vi "Check if Attribute is a Pointer.vi"(7 "Test ID":string, 8 "error in (no error)":errorcluster, 9 "Type":variant, 10 "Attribute Name":string, 11 "Test Executive in":refnum<class "Test Executive.lvclass">) -> (0 "error out":errorcluster, 1 "Pointer ID":string, 2 "Pointer?":bool, 3 "Test Executive out":refnum<class "Test Executive.lvclass">, 4 "Pointer Attribute Name":string)   [LabVIEW 2019, in "Test Executive.lvlib" / "Test Executive.lvclass"]
uses:
  <vilib>/gpm_packages/@cs/test-executive/Source/Test Executive/TestExecutive/Test Executive.lvclass
  <vilib>/gpm_packages/@cs/test-executive/Source/Test Executive/TestExecutive/Test Executive.lvclass/Test Executive.ctl
  67b02e64-984f-4c06-84dc-e4ea2e0dd7a9.vi
  <vilib>/gpm_packages/@cs/linked-list/Source/Linked List/ILinkedList/ILinked List.lvclass
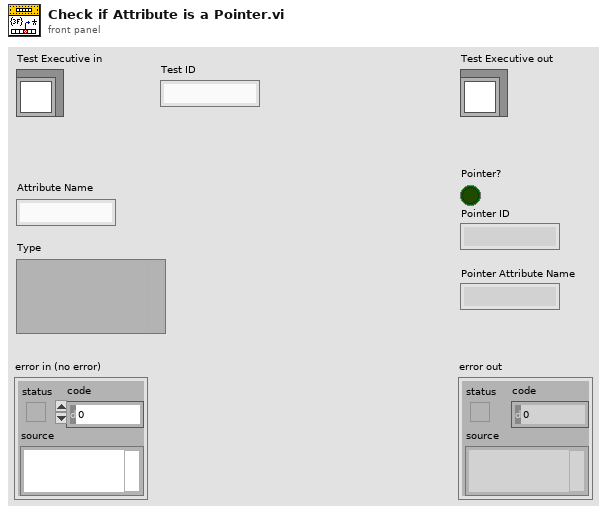
[diagram p1: front panel]
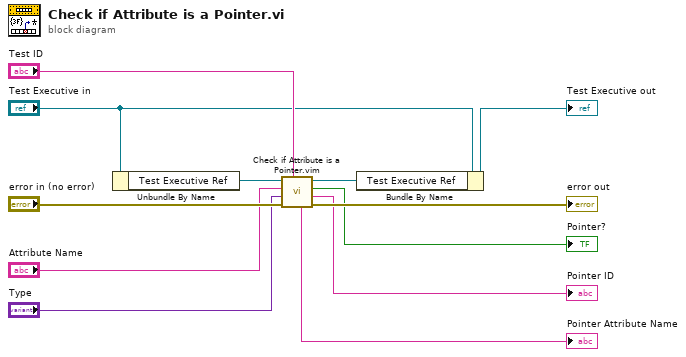
[diagram p0: block diagram]
diagram:
  n1 = Unbundle By Name("Test Executive in") -> ("Test Executive Ref"=w10:refnum<data-value>)
  n2 = call "Check if Attribute is a Pointer.vim"("Linked List ID"="Test ID", "error in (no error)"="error in (no error)", "Type"="Type", "Attribute Name"="Attribute Name", "Linked List Ref"=w10) -> ("error out"=→"error out":errorcluster, "Pointer ID"=→"Pointer ID":string, "Pointer?"=→"Pointer?":bool, "Linked List Ref out"=w8:refnum<data-value>, "Pointer Attribute Name"=→"Pointer Attribute Name":string)  [unwired: 2 in]
  n3 = Bundle By Name(cluster="Test Executive in", "Test Executive Ref"=w8) -> (→"Test Executive out":refnum<class "Test Executive.lvclass">)
